vi "FGV PWM.vi"(8 "error in (no error)":errorcluster caption="Fehler (Eingang, kein Fehler)") -> (0 "error out":errorcluster caption="Fehler (Ausgang)")   [LabVIEW 2020, in "Regler.lvlib"]
uses:
  Regler.lvlib
  FGV Daten Regler Aktionen.ctl
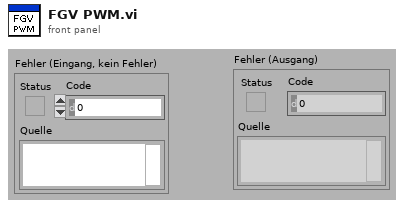
[diagram p1: front panel]
types:
  T1 = typedef "Regler.lvlib/FGV Daten Regler Aktionen.ctl" = enum16{"lesen", "Out%", "Heizung EIN"}
  T2 = cluster{"Output% 1":i16, "Output% 2":i16, "Output% 3":i16, "Output% 4":i16, "Output% 5":i16, "Output% 6":i16, "Output% 7":i16, "Output% 8":i16, "Output% 9":i16, "Output% 10":i16, "Output% 11":i16, "Output% 12":i16, "Output% 13":i16, "Output% 14":i16, "Output% 15":i16, "Output% 16":i16, "Output% 17":i16, "Output% 18":i16}
  T3 = cluster{"Output% 1":sgl, "Output% 2":sgl, "Output% 3":sgl, "Output% 4":sgl, "Output% 5":sgl, "Output% 6":sgl, "Output% 7":sgl, "Output% 8":sgl, "Output% 9":sgl, "Output% 10":sgl, "Output% 11":sgl, "Output% 12":sgl, "Output% 13":sgl, "Output% 14":sgl, "Output% 15":sgl, "Output% 16":sgl, "Output% 17":sgl, "Output% 18":sgl}
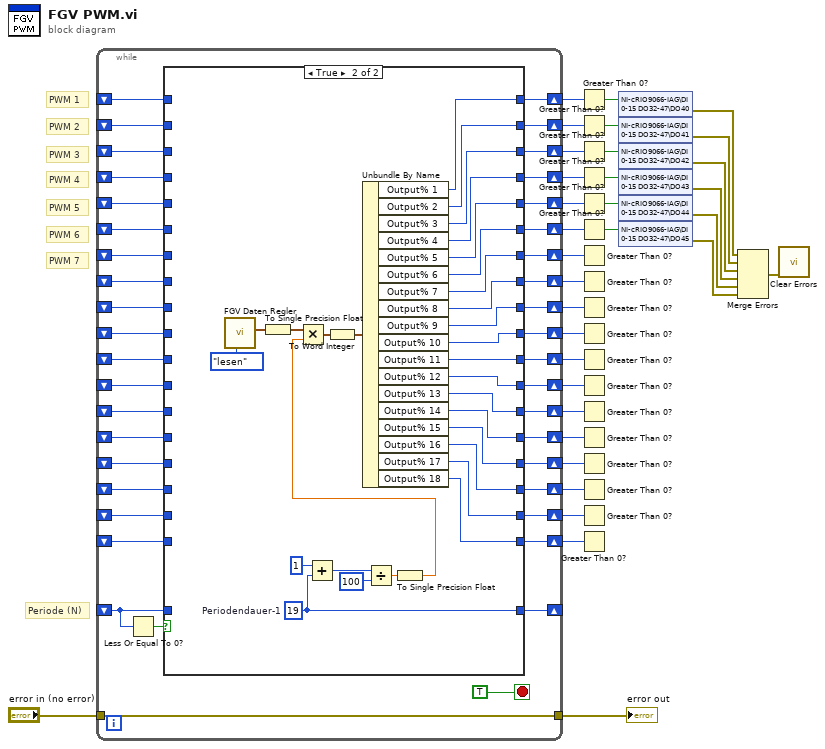
[diagram p0: block diagram]
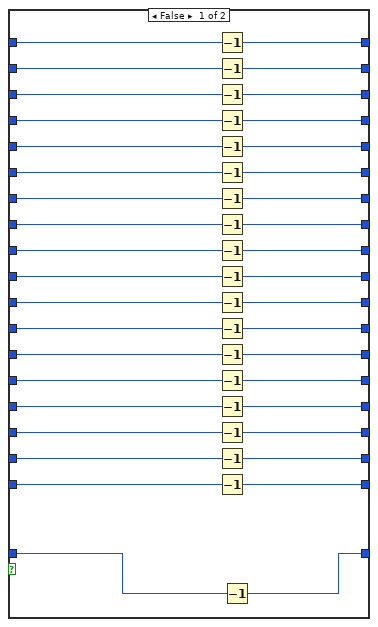
[diagram p2: hidden frame]
diagram:
  # "PWM 7"
  # "PWM 6"
  # "PWM 5"
  # "PWM 4"
  # "Periode (N)"
  # "PWM 3"
  # "PWM 2"
  # "PWM 1"
  n1 = while {
    shift-right: [w71] -> w33
    shift-left: _ -> [w64]
    shift-right: [w70] -> w32
    shift-left: _ -> [w63]
    shift-right: [w72] -> _
    shift-left: _ -> [w65]
    shift-right: [w69] -> w28
    shift-left: _ -> [w62]
    shift-right: [w68] -> w31
    shift-left: _ -> [w61]
    shift-right: [w67] -> w30
    shift-left: _ -> [w60]
    shift-right: [w66] -> w29
    shift-left: _ -> [w59]
    shift-right: [w58] -> w27
    shift-left: _ -> [w57]
    shift-right: [w56] -> w26
    shift-left: _ -> [w51]
    shift-right: [w55] -> w25
    shift-left: _ -> [w50]
    shift-right: [w54] -> w24
    shift-left: _ -> [w49]
    shift-right: [w53] -> w23
    shift-left: _ -> [w48]
    shift-right: [w52] -> w20
    shift-left: _ -> [w47]
    tunnel: "error in (no error)" -> [w46]
    tunnel: [w46] -> w21
    shift-right: [w45] -> w18
    shift-left: _ -> [w39]
    shift-right: [w43] -> w11
    shift-left: _ -> [w38]
    shift-right: [w42] -> w10
    shift-left: _ -> [w37]
    shift-right: [w41] -> w9
    shift-left: _ -> [w36]
    shift-right: [w40] -> w8
    shift-left: _ -> [w35]
    shift-right: [w44] -> w17
    shift-left: _ -> [w34]
    stop <- TRUE stop-if-true
    n2 = Less Or Equal To 0?(x=w65) -> (x <= 0?=w73:bool)
    n3 = case shown="True" w73 {
      tunnel: [w100 w138] -> w72
      tunnel: w65 -> [w101 _]
      tunnel: [w106 w137] -> w71
      tunnel: [w105 w136] -> w70
      tunnel: [w104 w135] -> w69
      tunnel: [w103 w134] -> w68
      tunnel: [w102 w133] -> w67
      tunnel: [w99 w132] -> w66
      tunnel: w64 -> [w112 _]
      tunnel: w63 -> [w111 _]
      tunnel: w62 -> [w110 _]
      tunnel: w61 -> [w109 _]
      tunnel: w60 -> [w108 _]
      tunnel: w59 -> [w107 _]
      tunnel: [w98 w131] -> w58
      tunnel: w57 -> [w97 _]
      tunnel: [w94 w128] -> w56
      tunnel: [w93 w118] -> w55
      tunnel: [w88 w127] -> w54
      tunnel: [w87 w126] -> w53
      tunnel: [w95 w125] -> w52
      tunnel: w51 -> [w92 _]
      tunnel: w50 -> [w91 _]
      tunnel: w49 -> [w90 _]
      tunnel: w48 -> [w89 _]
      tunnel: w47 -> [w96 _]
      tunnel: [w86 w124] -> w45
      tunnel: [w85 w119] -> w44
      tunnel: [w84 w123] -> w43
      tunnel: [w83 w122] -> w42
      tunnel: [w82 w121] -> w41
      tunnel: [w81 w120] -> w40
      tunnel: w39 -> [w80 _]
      tunnel: w38 -> [w79 _]
      tunnel: w37 -> [w78 _]
      tunnel: w36 -> [w77 _]
      tunnel: w35 -> [w76 _]
      tunnel: w34 -> [w75 _]
      frame False {
        n4 = Decrement(x=w112) -> (x-1=w106:i16)
        n5 = Decrement(x=w111) -> (x-1=w105:i16)
        n6 = Decrement(x=w110) -> (x-1=w104:i16)
        n7 = Decrement(x=w109) -> (x-1=w103:i16)
        n8 = Decrement(x=w108) -> (x-1=w102:i16)
        n9 = Decrement(x=w107) -> (x-1=w99:i16)
        n10 = Decrement(x=w97) -> (x-1=w98:i16)
        n11 = Decrement(x=w92) -> (x-1=w94:i16)
        n12 = Decrement(x=w91) -> (x-1=w93:i16)
        n13 = Decrement(x=w90) -> (x-1=w88:i16)
        n14 = Decrement(x=w89) -> (x-1=w87:i16)
        n15 = Decrement(x=w96) -> (x-1=w95:i16)
        n16 = Decrement(x=w80) -> (x-1=w86:i16)
        n17 = Decrement(x=w79) -> (x-1=w84:i16)
        n18 = Decrement(x=w78) -> (x-1=w83:i16)
        n19 = Decrement(x=w77) -> (x-1=w82:i16)
        n20 = Decrement(x=w76) -> (x-1=w81:i16)
        n21 = Decrement(x=w75) -> (x-1=w85:i16)
        n22 = Decrement(x=w101) -> (x-1=w100:i16)
      }
      frame True {
        w138 = i16 19  # Periodendauer-1
        n23 = call "FGV Daten Regler.vi"("Aktionen"=FGV_Daten_Regler_Aktionen."lesen") -> ("PID - OUT%"=w114:T2)  [unwired: 9 in, 1 out]
        n24 = To Single Precision Float(number=w114) -> (single precision float=w113:T3)
        n25 = Add(x=i16 1, y=w138) -> (x+y=w140:i16)
        n26 = Divide(x=w140, y=i16 100) -> (x/y=w117:dbl)
        n27 = To Single Precision Float(number=w117) -> (single precision float=w116:sgl)
        n28 = Multiply(x=w113, y=w116) -> (x*y=w130:T3)
        n29 = To Word Integer(number=w130) -> (16bit integer=w129:T2)
        n30 = Unbundle By Name(w129) -> ("Output% 1"=w137:i16, "Output% 2"=w136:i16, "Output% 3"=w135:i16, "Output% 4"=w134:i16, "Output% 5"=w133:i16, "Output% 6"=w132:i16, "Output% 7"=w131:i16, "Output% 8"=w128:i16, "Output% 9"=w118:i16, "Output% 10"=w127:i16, "Output% 11"=w126:i16, "Output% 12"=w125:i16, "Output% 13"=w124:i16, "Output% 14"=w123:i16, "Output% 15"=w122:i16, "Output% 16"=w121:i16, "Output% 17"=w120:i16, "Output% 18"=w119:i16)
      }
    }
  }
  "error out" <- w21
  n31 = Greater Than 0?(x=w33) -> (x > 0?=w19:bool)
  n32 = Greater Than 0?(x=w32) -> (x > 0?=w16:bool)
  n33 = Greater Than 0?(x=w28) -> (x > 0?=w15:bool)
  n34 = Greater Than 0?(x=w31) -> (x > 0?=w14:bool)
  n35 = Greater Than 0?(x=w30) -> (x > 0?=w13:bool)
  n36 = Greater Than 0?(x=w29) -> (x > 0?=w12:bool)
  n37 = Greater Than 0?(x=w27) -> ()  [unwired: 1 out]
  n38 = Greater Than 0?(x=w26) -> ()  [unwired: 1 out]
  n39 = Greater Than 0?(x=w25) -> ()  [unwired: 1 out]
  n40 = Greater Than 0?(x=w24) -> ()  [unwired: 1 out]
  n41 = Greater Than 0?(x=w23) -> ()  [unwired: 1 out]
  n42 = Greater Than 0?(x=w20) -> ()  [unwired: 1 out]
  n43 = Greater Than 0?(x=w18) -> ()  [unwired: 1 out]
  n44 = Greater Than 0?(x=w11) -> ()  [unwired: 1 out]
  n45 = Greater Than 0?(x=w10) -> ()  [unwired: 1 out]
  n46 = Greater Than 0?(x=w9) -> ()  [unwired: 1 out]
  n47 = Greater Than 0?(x=w8) -> ()  [unwired: 1 out]
  n48 = Greater Than 0?(x=w17) -> ()  [unwired: 1 out]
  n49 = shared-variable "NI-cRIO9066-IAG\\DI 0-15 DO32-47\\DO40"(w19) -> (error out=w6:errorcluster)  [unwired: 1 in]
  n50 = shared-variable "NI-cRIO9066-IAG\\DI 0-15 DO32-47\\DO41"(w16) -> (error out=w5:errorcluster)  [unwired: 1 in]
  n51 = shared-variable "NI-cRIO9066-IAG\\DI 0-15 DO32-47\\DO42"(w15) -> (error out=w4:errorcluster)  [unwired: 1 in]
  n52 = shared-variable "NI-cRIO9066-IAG\\DI 0-15 DO32-47\\DO43"(w14) -> (error out=w3:errorcluster)  [unwired: 1 in]
  n53 = shared-variable "NI-cRIO9066-IAG\\DI 0-15 DO32-47\\DO44"(w13) -> (error out=w2:errorcluster)  [unwired: 1 in]
  n54 = shared-variable "NI-cRIO9066-IAG\\DI 0-15 DO32-47\\DO45"(w12) -> (error out=w1:errorcluster)  [unwired: 1 in]
  n55 = Merge Errors(w6, w5, w4, w3, w2, w1) -> (w7:errorcluster)
  n56 = call <vilib>:"Clear Errors.vi"("error in (no error)"=w7) -> ()  [unwired: 5 in, 2 out]
